vi "Write Stop Notifier.vi"(8 "error in (no error)":errorcluster, 10 "Stop Notifier":refnum<notifier>, 11 "GUI in":refnum<class "GUI.lvclass">) -> (0 "error out":errorcluster, 3 "GUI out":refnum<class "GUI.lvclass">)   [LabVIEW 2012, in "GUI.lvclass"]
uses:
  GUI.lvclass
  GUI.lvclass/GUI.ctl
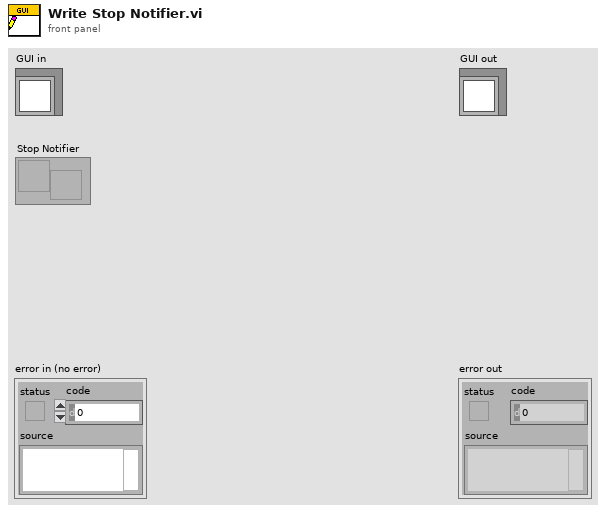
[diagram p1: front panel]
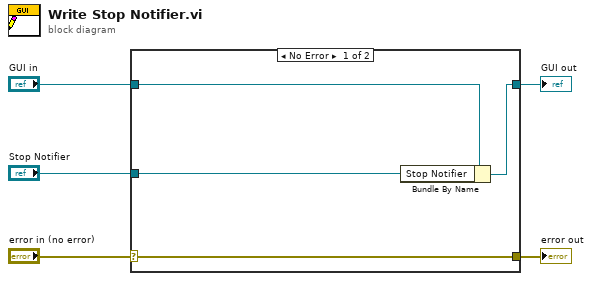
[diagram p0: block diagram]
diagram:
  n1 = case shown="No Error" "error in (no error)" {
    selector: "error in (no error)" -> [w9 w10]
    tunnel: [w9 w10] -> w4
    tunnel: [w7 w11] -> w2
    tunnel: "GUI in" -> [w8 w11]
    tunnel: "Stop Notifier" -> [w6 _]
    frame No Error {
      n2 = Bundle By Name(cluster=w8, "Stop Notifier"=w6) -> (w7:refnum<class "GUI.lvclass">)
    }
    frame Error {
    }
  }
  "error out" <- w4
  "GUI out" <- w2
